vi "Test.vi"() -> ()   [LabVIEW 2011, in "Owlstone GEN-SYS.lvclass"]
uses:
  Owlstone GEN-SYS.lvclass
  GEN-SYS Connections.ctl
  Michell Easidew/Michell Easidew.lvclass
  Eurotherm 3200 PID Controller/Eurotherm 3200 PID Controller.lvclass
  Permeation Tube.ctl
  Permeation Tube Gas.ctl
  Gen-Sys Setpoints.ctl
  Vapour Generator/Gas Output.ctl
  Vapour Generator/Vapour Generator.lvclass
panel:
  out "Gas Output":T1={"Concentration (ppm)"=20.928351576786866, "Flow Rate (ml/min)"=100.0, "Relative Humidity (%)"=1.2743154039806512} {"Relative Humidity (%)" format="%#.4g"; "Flow Rate (ml/min)" format="%#.0f"; "Concentration (ppm)" format="%#.2g"}
  in  "stop":bool
  in  "Setpoints":T2={"OVG-4"={"Oven Temperature"=70, "Sample Flow Rate"=100, "Split Flow Status"=0, "Split Flow Rate"=1000}, "OHG-4"={"Wet Air Flow"=600}} {"OHG-4"."Wet Air Flow" min=300 max=3000 scale=300.0..3000.0; "OVG-4"."Split Flow Status" items=["Closed", "Open"]; "OVG-4"."Split Flow Rate" min=300 max=3000 scale=50.0..3000.0; "OVG-4"."Sample Flow Rate" min=50 max=500 scale=50.0..500.0; "OVG-4"."Oven Temperature" min=25 max=100 scale=25.0..100.0}
  in  "Permeation Tube":T3={"Tube"=enum."Isobutylene 27 Nov 2012", "Molecular Weight"=56.106, "Calibration Temperature\n(Celcius)"=50, "Permeation Rate \n(ng/min)"=1539} {"Molecular Weight" min=0.0 format="%#_3g"; "Permeation Rate \n(ng/min)" min=0; "Calibration Temperature\n(Celcius)" min=0}
  out "Owlstone OVG-4 out":refnum<class "Owlstone GEN-SYS.lvclass">
  in  "Owlstone GEN-SYS":refnum<class "Owlstone GEN-SYS.lvclass">
  out "error out":errorcluster={"status"=FALSE, "code"=1073676294, "source"="VISA Read in Michell Easidew.lvclass:Get Humidity.vi->Owlstone GEN-SYS.lvclass:Get Gas Output.vi->Owlstone GEN-SYS.lvclass:Test.vi"}
  in  "Connections":T5={"GEN-SYS VISA resource name"="GENSYS", "OVG-4"={"Flow Address"=4, "Temp Address"=3}, "OHG-4"={"Flow Address"=1, "Easydew VISA resource name"="COM6"}}
  in  "error in":errorcluster
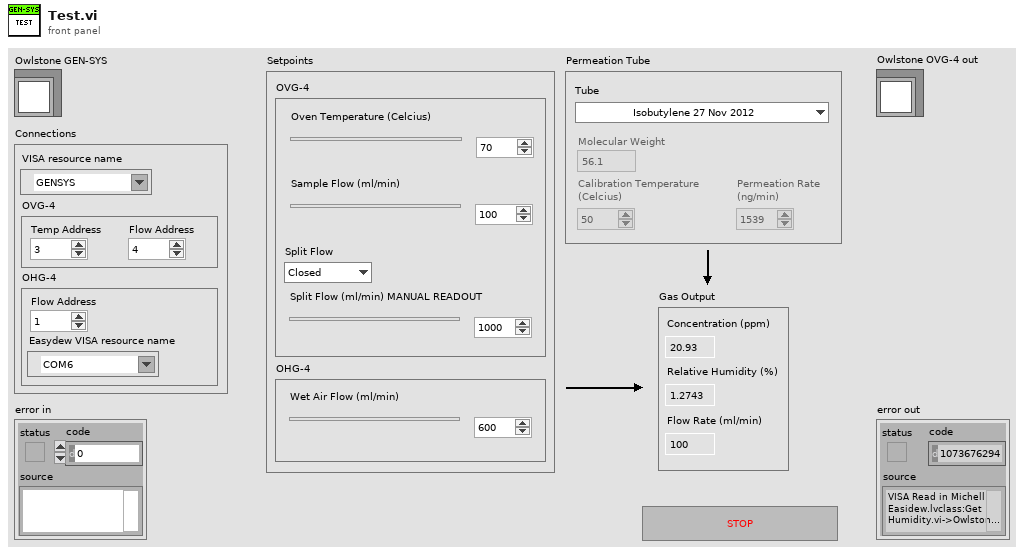
[diagram p1: front panel]
types:
  T1 = typedef "Vapour Generator.lvclass/Gas Output.ctl" = cluster{"Concentration (ppm)":dbl, "Flow Rate (ml/min)":dbl, "Relative Humidity (%)":dbl}
  T2 = typedef "Owlstone GEN-SYS.lvclass/Gen-Sys Setpoints.ctl" = cluster{"OVG-4":cluster{"Oven Temperature":i32, "Sample Flow Rate":i32, "Split Flow Status":u16, "Split Flow Rate":i32}, "OHG-4":cluster{"Wet Air Flow":i32}}
  T3 = typedef "Owlstone GEN-SYS.lvclass/Permeation Tube.ctl" = cluster{"Tube":T4, "Molecular Weight":dbl, "Calibration Temperature\n(Celcius)":i32, "Permeation Rate \n(ng/min)":i32}
  T4 = typedef "Owlstone GEN-SYS.lvclass/Permeation Tube Gas.ctl" = enum16{"Isobutylene 27 Nov 2012", "Ammonia 29 Sep 2012", "DMMP Tube A 3 July 2014", "DMMP Tube B 3 July 2014"}
  T5 = typedef "Owlstone GEN-SYS.lvclass/GEN-SYS Connections.ctl" = cluster{"GEN-SYS VISA resource name":refnum<visa-resource-name>, "OVG-4":cluster{"Flow Address":u8, "Temp Address":u8}, "OHG-4":cluster{"Flow Address":u8, "Easydew VISA resource name":refnum<visa-resource-name>}}
  T6 = enum8{"Enabled", "Disabled", "Disabled and Grayed Out"}
  T7 = cluster{"OVG-4":cluster{"Oven Temperature":i32, "Sample Flow Rate":i32, "Split Flow Status":u16, "Split Flow Rate":i32}, "OHG-4":cluster{"Wet Air Flow":i32}}
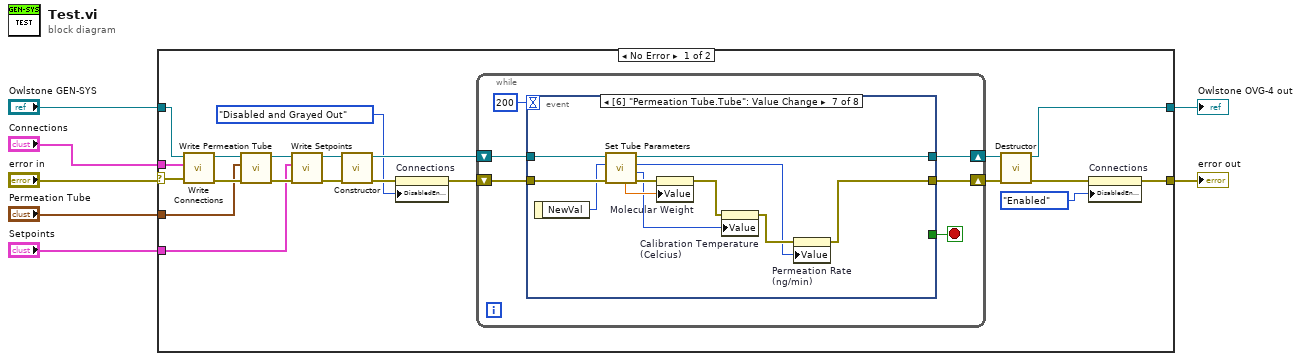
[diagram p0: block diagram]
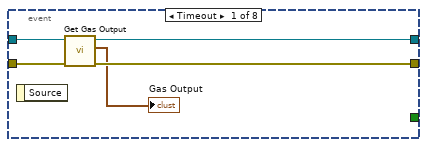
[diagram p2: hidden frame]
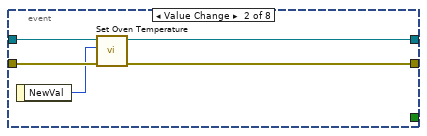
[diagram p3: hidden frame]
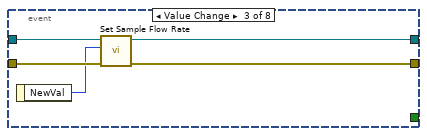
[diagram p4: hidden frame]
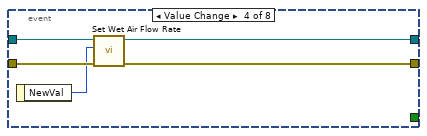
[diagram p5: hidden frame]
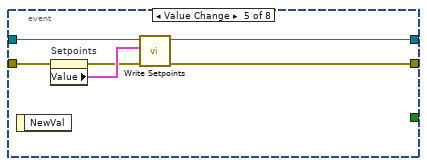
[diagram p6: hidden frame]
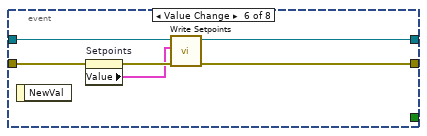
[diagram p7: hidden frame]
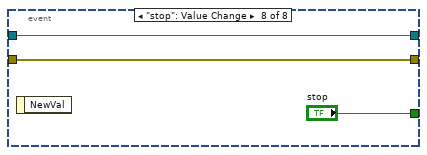
[diagram p8: hidden frame]
diagram:
  n1 = case shown="No Error" "error in" {
    selector: "error in" -> [w16 w80]
    tunnel: "Owlstone GEN-SYS" -> [w27 w81]
    tunnel: [w9 w80] -> w6
    tunnel: [w26 w81] -> w5
    tunnel: "Connections" -> [w25 _]
    tunnel: "Permeation Tube" -> [w18 _]
    tunnel: "Setpoints" -> [w17 _]
    frame No Error {
      n2 = call-dynamic "Write Connections.vi"("error in (no error)"=w16, "Connections"=w25, "Owlstone OVG-4 in"=w27) -> ("error out"=w23:errorcluster, "Owlstone OVG-4 out"=w24:refnum<class "Owlstone GEN-SYS.lvclass">)  [unwired: 7 in]
      n3 = call-dynamic "Write Permeation Tube.vi"("error in (no error)"=w23, "Permeation Tube"=w18, "Owlstone GEN-SYS in"=w24) -> ("error out"=w22:errorcluster, "Owlstone GEN-SYS out"=w21:refnum<class "Owlstone GEN-SYS.lvclass">)  [unwired: 7 in]
      n4 = call-dynamic "Write Setpoints.vi"("error in (no error)"=w22, "Setpoints"=w17, "Owlstone GEN-SYS in"=w21) -> ("error out"=w19:errorcluster, "Owlstone GEN-SYS out"=w20:refnum<class "Owlstone GEN-SYS.lvclass">)  [unwired: 7 in]
      n5 = call-dynamic "Constructor.vi"("error in"=w19, "Owlstone Gen-SYS in"=w20) -> ("error out"=w12:errorcluster, "Owlstone GEN-SYS out"=w15:refnum<class "Owlstone GEN-SYS.lvclass">)  [unwired: 7 in, 1 out]
      n6 = property on="Connections" class="Clust (strict)"(error in=w12, "DisabledEnum"=T6."Disabled and Grayed Out" ("Disabled")) -> ()  [unwired: 1 in, 2 out]
      n7 = while {
        shift-right: [w30] -> w14
        shift-left: w15 -> [w32]
        shift-right: [w31] -> w13
        shift-left: w12 -> [w33]
        stop <- w29 stop-if-true
        n8 = event shown="[6] \"Permeation Tube.Tube\": Value Change" {
          selector: _ -> [_ _ _ _ _ _ _ _]
          dyn-events: _ -> [_ _ _ _ _ _ _ _]
          timeout: 200 -> [_ _ _ _ _ _ _ _]
          tunnel: w33 -> [w38 w42 w48 w53 w59 w62 w75 w77]
          tunnel: w32 -> [w37 w43 w47 w52 w56 w65 w76 w78]
          tunnel: [w35 w40 w44 w50 w54 w63 w67 w77] -> w31
          tunnel: [w36 w39 w45 w51 w55 w64 w74 w78] -> w30
          tunnel: [_ _ _ _ _ _ _ "stop"] -> w29
          event Timeout {
            n9 = event-data() -> ()  [unwired: 1 in, 1 out]
            n10 = call-dynamic "Get Gas Output.vi"("error in"=w38, "Owlstone OVG-4 in"=w37) -> ("error out"=w35:errorcluster, "Output"=→"Gas Output":T1, "Owlstone OVG-4 out"=w36:refnum<class "Owlstone GEN-SYS.lvclass">)  [unwired: 7 in]
          }
          event Value Change {
            n11 = event-data() -> ("NewVal"=w41:i32)  [unwired: 1 in]
            n12 = call "Set Oven Temperature.vi"("error in"=w42, "Oven Temperature"=w41, "OVG In"=w43) -> ("error out"=w40:errorcluster, "OVG Out"=w39:refnum<class "Owlstone GEN-SYS.lvclass">)  [unwired: 7 in]
          }
          event Value Change {
            n13 = event-data() -> ("NewVal"=w46:i32)  [unwired: 1 in]
            n14 = call "Set Sample Flow Rate.vi"("error in"=w48, "Sample Flow"=w46, "OVG In"=w47) -> ("error out"=w44:errorcluster, "OVG Out"=w45:refnum<class "Owlstone GEN-SYS.lvclass">)  [unwired: 7 in]
          }
          event Value Change {
            n15 = event-data() -> ("NewVal"=w49:i32)  [unwired: 1 in]
            n16 = call "Set Wet Air Flow Rate.vi"("error in"=w53, "Wet Air Flow Rate (ml/min)"=w49, "OVG In"=w52) -> ("error out"=w50:errorcluster, "OVG Out"=w51:refnum<class "Owlstone GEN-SYS.lvclass">)  [unwired: 7 in]
          }
          event Value Change {
            n17 = event-data() -> ()  [unwired: 1 in, 1 out]
            n18 = property on="Setpoints" class="Clust (strict)"(error in=w59) -> (error out=w57:errorcluster, "Value"=w58:T7)  [unwired: 1 in, 1 out]
            n19 = call-dynamic "Write Setpoints.vi"("error in (no error)"=w57, "Setpoints"=w58, "Owlstone GEN-SYS in"=w56) -> ("error out"=w54:errorcluster, "Owlstone GEN-SYS out"=w55:refnum<class "Owlstone GEN-SYS.lvclass">)  [unwired: 7 in]
          }
          event Value Change {
            n20 = event-data() -> ()  [unwired: 1 in, 1 out]
            n21 = property on="Setpoints" class="Clust (strict)"(error in=w62) -> (error out=w61:errorcluster, "Value"=w60:T7)  [unwired: 1 in, 1 out]
            n22 = call-dynamic "Write Setpoints.vi"("error in (no error)"=w61, "Setpoints"=w60, "Owlstone GEN-SYS in"=w65) -> ("error out"=w63:errorcluster, "Owlstone GEN-SYS out"=w64:refnum<class "Owlstone GEN-SYS.lvclass">)  [unwired: 7 in]
          }
          event Value Change {
            n23 = event-data() -> ("NewVal"=w66:T4)  [unwired: 1 in]
            n24 = call-dynamic "Set Tube Parameters.vi"("error in (no error)"=w75, "Tube Gas"=w66, "Owlstone GEN-SYS in"=w76) -> ("error out"=w73:errorcluster, "Calibration Temperature"=w71:i32, "Permeation Rate"=w68:i32, "Owlstone GEN-SYS out"=w74:refnum<class "Owlstone GEN-SYS.lvclass">, "Molecular Weight"=w72:dbl)  [unwired: 4 in]
            n25 = property on="Molecular Weight" class="DigNum (strict)"(error in=w73, "Value"=w72) -> (error out=w70:errorcluster)  [unwired: 1 in, 1 out]
            n26 = property on="Calibration Temperature\n(Celcius)" class="DigNum (strict)"(error in=w70, "Value"=w71) -> (error out=w69:errorcluster)  [unwired: 1 in, 1 out]
            n27 = property on="Permeation Rate \n(ng/min)" class="DigNum (strict)"(error in=w69, "Value"=w68) -> (error out=w67:errorcluster)  [unwired: 1 in, 1 out]
          }
          event "stop": Value Change {
            n28 = event-data() -> ()  [unwired: 1 in, 1 out]
          }
        }
      }
      n29 = call-dynamic "Destructor.vi"("error in"=w13, "Owlstone OVG-4 in"=w14) -> ("error out"=w10:errorcluster, "Owlstone OVG-4 out"=w26:refnum<class "Owlstone GEN-SYS.lvclass">)  [unwired: 8 in]
      n30 = property on="Connections" class="Clust (strict)"(error in=w10, "DisabledEnum"=T6."Enabled" ("Disabled")) -> (error out=w9:errorcluster)  [unwired: 1 in, 1 out]
    }
    frame Error {
    }
  }
  "error out" <- w6
  "Owlstone OVG-4 out" <- w5
